vi "DataReadGen.vi"(0 "error in":errorcluster, 2 "Index (0)":i64, 3 "chemin Data":path) -> (5 "DernColVal":i32, 6 "error out":errorcluster, 7 "LastScanPos":dbl[](array[numeric]), 8 "XY Graph":T1(array[cluster]), 9 "AllYData":dbl[][](array[numeric]) format="%#.3f")   [LabVIEW 2010]
doc: "Ce VI lit les données contenu dans le fichier de sauvegarde automatique. Ces données correspondent aux valeurs prises lors du dernier balayage. La sauvegarde automatique est effectué après chaque acquisition."
panel:
  out "LastScanPos 2":dbl[](array[numeric])
  out "AllYData 2":dbl[][](array[numeric]) format="%#_15f"
  in  "indice":i32
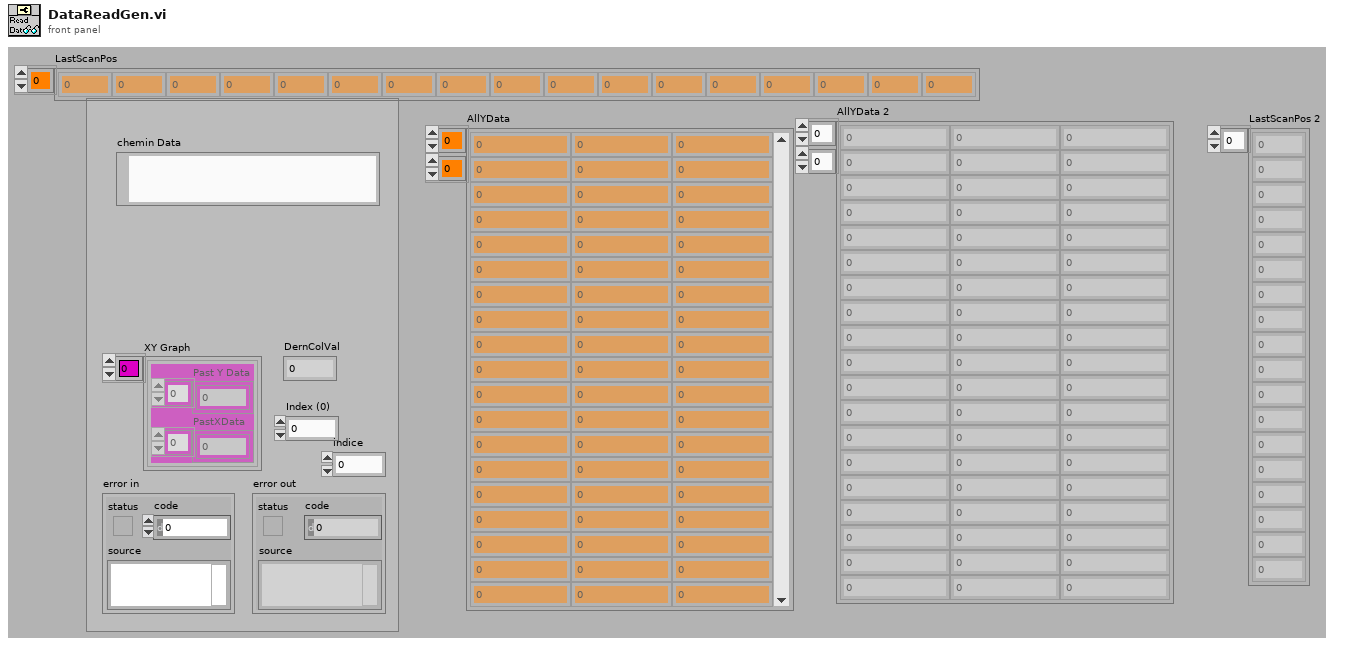
[diagram p1: front panel]
types:
  T1 = cluster{"Past Y Data":dbl[], "PastXData":dbl[]}[]
  T2 = cluster{"AllYData 2":dbl[][], "XY Graph":cluster{"Past Y Data":dbl[], "PastXData":dbl[]}[], "LastScanPos 2":dbl[]}
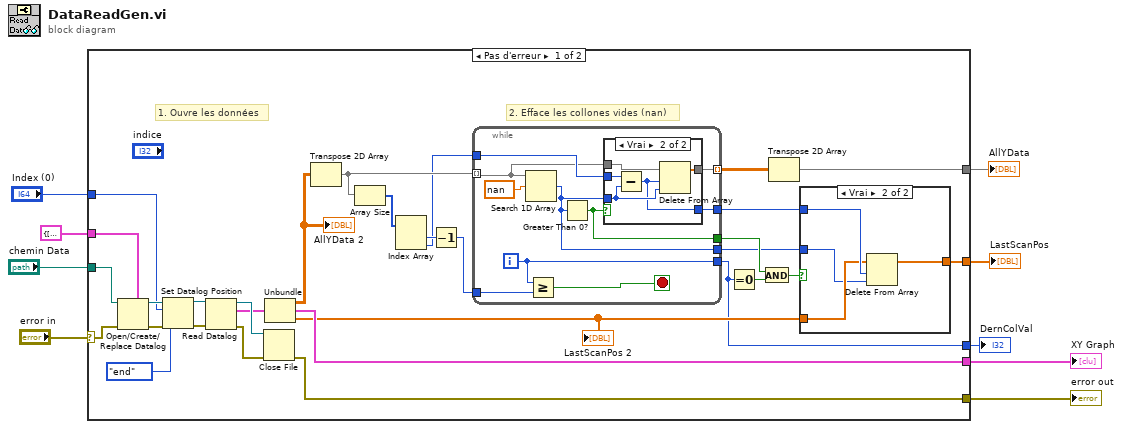
[diagram p0: block diagram]
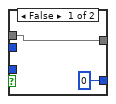
[diagram p3: hidden frame]
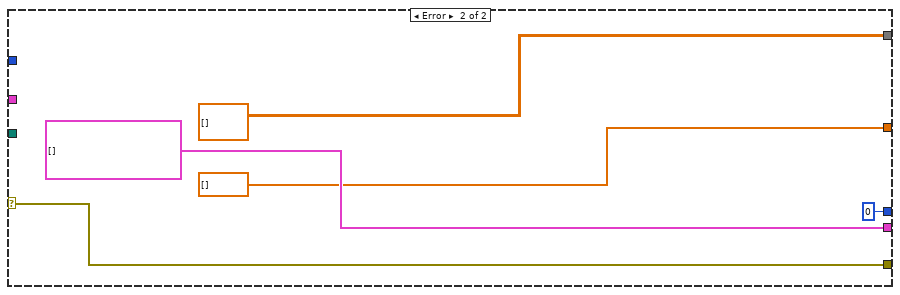
[diagram p4: hidden frame]
diagram:
  n1 = case shown="Pas d'erreur" "error in" {
    selector: "error in" -> [w35 w63]
    tunnel: "chemin Data" -> [w39 _]
    tunnel: T2 {"AllYData 2"=[], "XY Graph"=[], "LastScanPos 2"=[]} ("output cluster") -> [w38 _]
    tunnel: [w34 w63] -> w8
    tunnel: [w23 dbl[][] [] ("AllYData 2")] -> w7
    tunnel: [w36 T1 [] ("XY Graph")] -> w4
    tunnel: [w26 dbl[] [] ("LastScanPos 2")] -> w6
    tunnel: [w18 0] -> w3
    tunnel: "Index (0)" -> [w12 _]
    frame No Error {
      # "2. Efface les collones vides (nan)"
      # "1. Ouvre les données"
      n2 = Open/Create/Replace Datalog(5:w38, 8:w35, 11:w39) -> (0:w14:errorcluster, 3:w15:refnum<k1>)  [unwired: 3 in, 1 out]
      n3 = Set Datalog Position(4:w14, 5:enum16{"start", "end", "current"}."end" ("à partir de (0 : start)"), 6:w12, 7:w15) -> (0:w13:errorcluster, 3:w16:refnum<k1>)
      n4 = Read Datalog(4:w13, 7:w16) -> (0:w37:errorcluster, 2:w10:T2, 3:w33:refnum<k1>)  [unwired: 1 in]
      n5 = Close File(refnum=w33, error in=w37) -> (error out=w34:errorcluster)  [unwired: 1 out]
      n6 = Unbundle(w10) -> ("AllYData 2"=w27:dbl[][], "XY Graph"=w36:T1, "LastScanPos 2"=w28:dbl[])
      "AllYData 2" <- w27
      "LastScanPos 2" <- w28
      n7 = Transpose 2D Array(2D array=w27) -> (transposed array=w29:dbl[][])
      n8 = Array Size(array=w29) -> (size(s)=w32:i32[])
      n9 = Index Array(array=w32) -> (element #1=w31:i32, element #2=w25:i32)  [unwired: 2 in]
      n10 = Decrement(x=w31) -> (x-1=w30:i32)
      n11 = while {
        tunnel: w29 -> [w50] mode=indexing
        tunnel: [w52] -> w18
        tunnel: w30 -> [w53]
        tunnel: w25 -> [w51]
        tunnel: [w49] -> w24 mode=indexing
        tunnel: [w48] -> w17
        tunnel: [w46] -> w21
        tunnel: [w47] -> w19
        i -> [w52]
        stop <- w45 stop-if-true
        n12 = Search 1D Array(1D array=w50, element=nan ("élément")) -> (index of element=w48:i32)  [unwired: 1 in]
        n13 = Greater Or Equal?(x=w52, y=w53) -> (x >= y?=w45:bool)
        n14 = Greater Than 0?(x=w48) -> (x > 0?=w46:bool)
        n15 = case shown="Vrai" w46 {
          tunnel: w51 -> [_ w61]
          tunnel: w48 -> [_ w59]
          tunnel: w50 -> [w56 w60]
          tunnel: [w56 w58] -> w49
          tunnel: [0 w57] -> w47
          frame False {
          }
          frame True {
            n16 = Subtract(x=w61, y=w59) -> (x-y=w57:i32)
            n17 = Delete From Array(array=w60, length=w57, index=w59) -> (array with subset deleted=w58:dbl[])  [unwired: 1 out]
          }
        }
      }
      n18 = Equal To 0?(x=w18) -> (x = 0?=w22:bool)
      n19 = And(x=w21, y=w22) -> (x .and. y?=w20:bool)
      n20 = Transpose 2D Array(2D array=w24) -> (transposed array=w23:dbl[][])
      n21 = case shown="Vrai" w20 {
        tunnel: w28 -> [w40 w43]
        tunnel: [w40 w42] -> w26
        tunnel: w19 -> [_ w44]
        tunnel: w17 -> [_ w41]
        frame False {
        }
        frame True {
          n22 = Delete From Array(array=w43, length=w44, index=w41) -> (array with subset deleted=w42:dbl[])  [unwired: 1 out]
        }
      }
    }
    frame Error {
    }
  }
  "error out" <- w8
  "AllYData" <- w7
  "LastScanPos" <- w6
  "XY Graph" <- w4
  "DernColVal" <- w3
